vi "SMU Reset.vi"(8 "error in (no error)":errorcluster, 9 "Remote Node (1)":i32=1, 10 "Reset Module (0: Entire System)":i32(ring) items=["Entire System", "Local Group", "Local Node", "Remote Node", "Source Measure Unit Channel A", "Source Measure Unit Channel B", "LAN", "TSP Net", "TSP Link", "Timer"], 11 "VISA resource name":refnum<visa-resource-name>) -> (0 "error out":errorcluster, 3 "VISA resource name out":refnum<visa-resource-name>)   [LabVIEW 2020, in "Keithley 2600 Series.lvlib"]
doc: "Recalls factory default setting."
uses:
  Keithley 2600 Series.lvlib
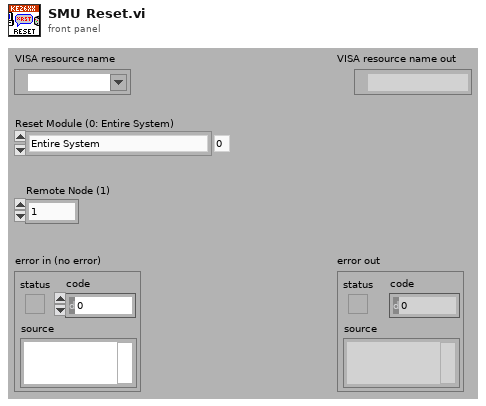
[diagram p1: front panel]
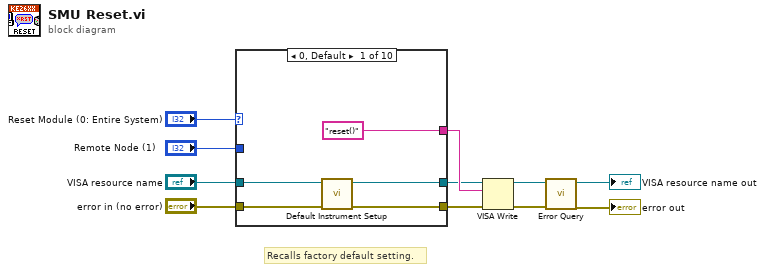
[diagram p0: block diagram]
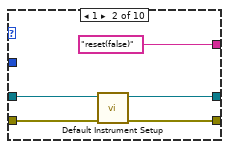
[diagram p2: hidden frame]
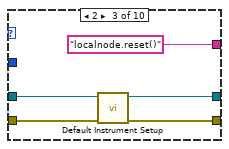
[diagram p3: hidden frame]
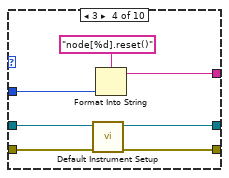
[diagram p4: hidden frame]
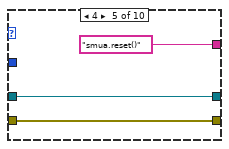
[diagram p5: hidden frame]
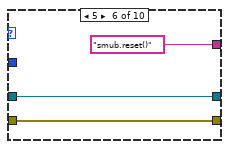
[diagram p6: hidden frame]
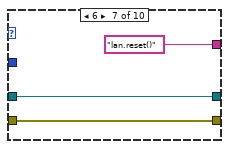
[diagram p7: hidden frame]
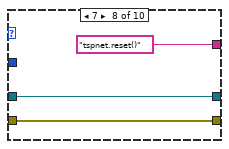
[diagram p8: hidden frame]
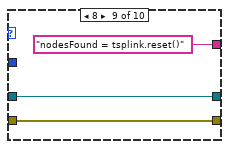
[diagram p9: hidden frame]
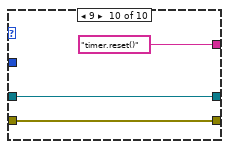
[diagram p10: hidden frame]
diagram:
  # "Recalls factory default setting."
  n1 = case shown="0, Default" "Reset Module (0: Entire System)" {
    tunnel: ["reset()" "reset(false)" "localnode.reset()" w33 "smua.reset()" "smub.reset()" "lan.reset()" "tspnet.reset()" "nodesFound = tsplink.reset()" "timer.reset()"] -> w6
    tunnel: "Remote Node (1)" -> [_ _ _ w31 _ _ _ _ _ _]
    tunnel: "VISA resource name" -> [w12 w20 w25 w30 w35 w38 w41 w44 w47 w50]
    tunnel: "error in (no error)" -> [w15 w19 w24 w29 w34 w37 w40 w43 w46 w49]
    tunnel: [w14 w18 w23 w28 w35 w38 w41 w44 w47 w50] -> w2
    tunnel: [w13 w17 w22 w27 w34 w37 w40 w43 w46 w49] -> w1
    frame 0, Default {
      n2 = call "Default Instrument Setup.vi"("error in (no error)"=w15, "VISA resource name"=w12) -> ("error out"=w13:errorcluster, "VISA resource name out"=w14:refnum<visa-resource-name>)  [unwired: 8 in]
    }
    frame 1 {
      n3 = call "Default Instrument Setup.vi"("error in (no error)"=w19, "VISA resource name"=w20) -> ("error out"=w17:errorcluster, "VISA resource name out"=w18:refnum<visa-resource-name>)  [unwired: 8 in]
    }
    frame 2 {
      n4 = call "Default Instrument Setup.vi"("error in (no error)"=w24, "VISA resource name"=w25) -> ("error out"=w22:errorcluster, "VISA resource name out"=w23:refnum<visa-resource-name>)  [unwired: 8 in]
    }
    frame 3 {
      n5 = call "Default Instrument Setup.vi"("error in (no error)"=w29, "VISA resource name"=w30) -> ("error out"=w27:errorcluster, "VISA resource name out"=w28:refnum<visa-resource-name>)  [unwired: 8 in]
      n6 = Format Into String(format string="node[%d].reset()", w31) -> (resulting string=w33:string)  [unwired: 2 in, 1 out]
    }
    frame 4 {
    }
    frame 5 {
    }
    frame 6 {
    }
    frame 7 {
    }
    frame 8 {
    }
    frame 9 {
    }
  }
  n7 = VISA Write(VISA resource name=w2, write buffer=w6, error in (no error)=w1) -> (VISA resource name out=w11:refnum<visa-resource-name>, error out=w10:errorcluster)  [unwired: 1 out]
  n8 = call "Error Query.vi"("error in (no error)"=w10, "VISA resource name"=w11) -> ("error out"=→"error out":errorcluster, "VISA resource name out"=→"VISA resource name out":refnum<visa-resource-name>)  [unwired: 6 in, 2 out]
